vi "Translator.TranslateThis.vi"(7 "Language (English)":string="English", 8 "error in":errorcluster, 11 "vi reference":refnum<vi>) -> (0 "error out":errorcluster)   [LabVIEW 2016]
uses:
  Global/ApplicationGlobal.vi
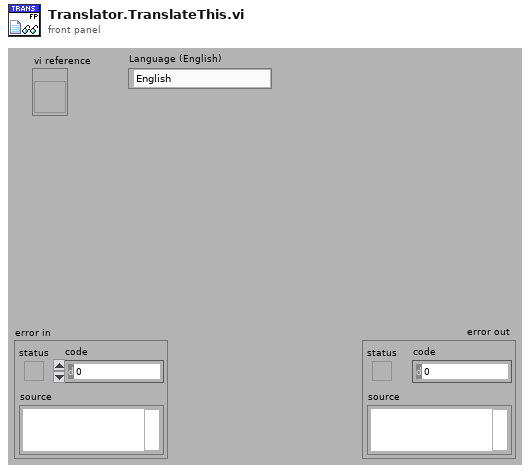
[diagram p1: front panel]
types:
  T1 = typedef "Translator.ControlData.ctl" = cluster{"ref":refnum<vi>, "strict?":bool, "save font?":bool, "type":T2, "root":string, "label":string, "caption":string, "bln.false":string, "bln.true":string, "cols":string[], "rows":string[]}
  T2 = typedef "Translator.ControlTypes.ctl" = enum16{"Cluster", "Array", "Boolean", "Ring", "String", "Tab", "Listbox", "Multicolumn listbox", "Table", "Tree", "Other"}
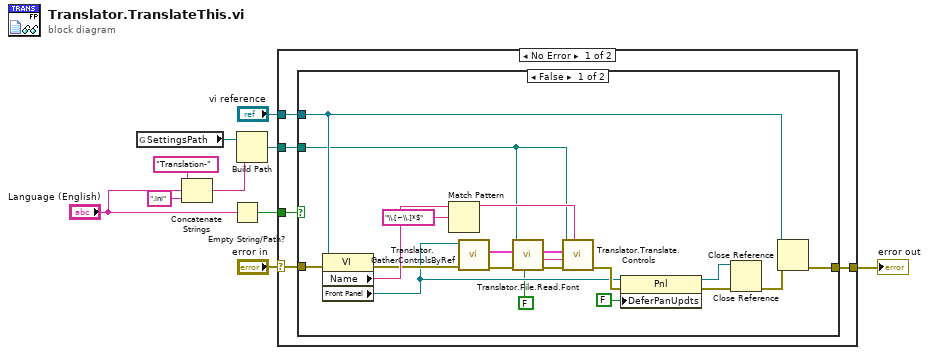
[diagram p0: block diagram]
diagram:
  n1 = global read "ApplicationGlobal.vi" "SettingsPath"() -> (w5:path)
  n2 = Concatenate Strings("Translation-" ("string"), "Language (English)", ".ini" ("string")) -> (w6:string)
  n3 = Empty String/Path?(string/path="Language (English)") -> (empty?=w1:bool)
  n4 = Build Path(base path=w5, name or relative path=w6) -> (appended path=w4:path)
  n5 = case shown="No Error" "error in" {
    selector: "error in" -> [w15 w36]
    tunnel: w4 -> [w12 _]
    tunnel: "vi reference" -> [w13 _]
    tunnel: [w14 w36] -> w8
    tunnel: w1 -> [w11 _]
    frame No Error {
      n6 = case shown="False" w11 {
        tunnel: w15 -> [w32 w35]
        tunnel: [w27 w35] -> w14
        tunnel: w13 -> [w23 _]
        tunnel: w12 -> [w21 _]
        frame False {
          n7 = property class="VI"(reference=w23, error in=w32) -> (error out=w18:errorcluster, "Name"=w26:string, "Front Panel"=w17:refnum<vi>)  [unwired: 1 out]
          n8 = Match Pattern(string=w26, regular expression="\\.[~\\.]*$") -> (before substring=w25:string)  [unwired: 4 out]
          n9 = call "Translator.GatherControlsByRef.vi"("error in"=w18, "Front Panel"=w17) -> ("error out"=w20:errorcluster, "Controls out"=w33:T1[])  [unwired: 8 in]
          n10 = call "Translator.File.Read.Font.vi"("Do not save font? (F)"=FALSE, "error in"=w20, "Translation file"=w21) -> ("error out"=w19:errorcluster, "font name"=w22:string)  [unwired: 6 in, 1 out]
          n11 = call "Translator.Translate.Controls.vi"("group"=w25, "error in"=w19, "font name"=w22, "Controls out"=w33, "Translation file"=w21) -> ("error out"=w24:errorcluster)  [unwired: 6 in]
          n12 = property class="Pnl"(reference=w17, error in=w24, "DeferPanUpdts"=FALSE ("Defer Panel Updates")) -> (reference out=w31:refnum<vi>, error out=w30:errorcluster)
          n13 = Close Reference(reference=w31, error in (no error)=w30) -> (error out=w28:errorcluster)
          n14 = Close Reference(reference=w23, error in (no error)=w28) -> (error out=w27:errorcluster)
        }
        frame True {
        }
      }
    }
    frame Error {
    }
  }
  "error out" <- w8
